vi "AppConfigTypeToXML.vi"(8 "error in (no error)":errorcluster, 11 "RingdownPlugin in":refnum<class "EraPlugin.lvclass">) -> (0 "error out":errorcluster, 2 "ConfigXML out":string, 3 "RingdownPlugin out":refnum<class "EraPlugin.lvclass">)   [LabVIEW 2017, in "AppPlugins.lvlib" / "ERAPlugin.lvclass"]
uses:
  EraPlugin.lvclass
  EraPlugin.lvclass/EraPlugin.ctl
  Accessors/Read RingdownConfig.vi
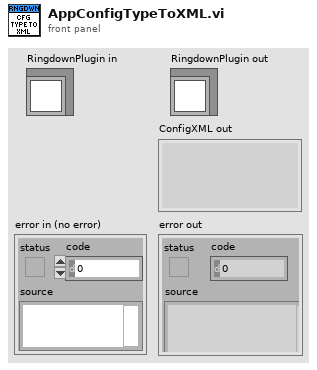
[diagram p1: front panel]
types:
  T1 = typedef "AppPlugins.lvlib/ERAPlugin.lvclass/RingdownConfig.ctl" = cluster{"Config":cluster{"p_SysOdr":i32, "dThres":dbl, "Preproc":cluster{"order":i32, "f_lo":dbl, "f_hi":dbl, "R_down":i32}}, "V index":i32, "I index":i32, "PosSeq":bool}
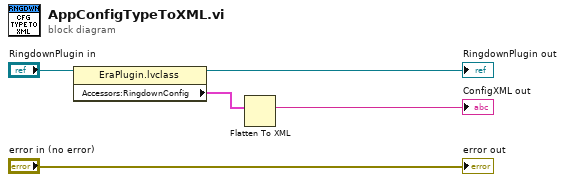
[diagram p0: block diagram]
diagram:
  n1 = property class="EraPlugin.lvclass"(reference="RingdownPlugin in") -> (reference out=→"RingdownPlugin out":refnum<class "EraPlugin.lvclass">, "Accessors:RingdownConfig"=w4:T1)  [unwired: 1 in, 1 out]
  n2 = Flatten To XML(anything=w4) -> (xml string=→"ConfigXML out":string)
  "error out" <- "error in (no error)"
